vi "component orientation check.vi"(8 "error in":errorcluster, 10 "input cluster":T1, 11 "Gantry In":refnum<k24>) -> (0 "error out":errorcluster, 1 "Wrong Orientation?":bool, 2 "output cluster":T1, 3 "Gantry Out":refnum<k24>)   [LabVIEW 2021, in "Component Tray.lvclass"]
uses:
  Component Tray.lvclass
  Find Component.ctl
  Controller/Camera/Machine Vision.ctl
  C:/Program Files (x86)/Aerotech/A3200/LabVIEW/2010/Bin/Aerotech.A3200.dll
  Program Files (x86)/Aerotech/A3200/LabVIEW/2010/Bin/Aerotech.A3200.dll
  Controller/Motion/A3200/A3200.lvclass
  Controller/Camera/Camera.lvclass
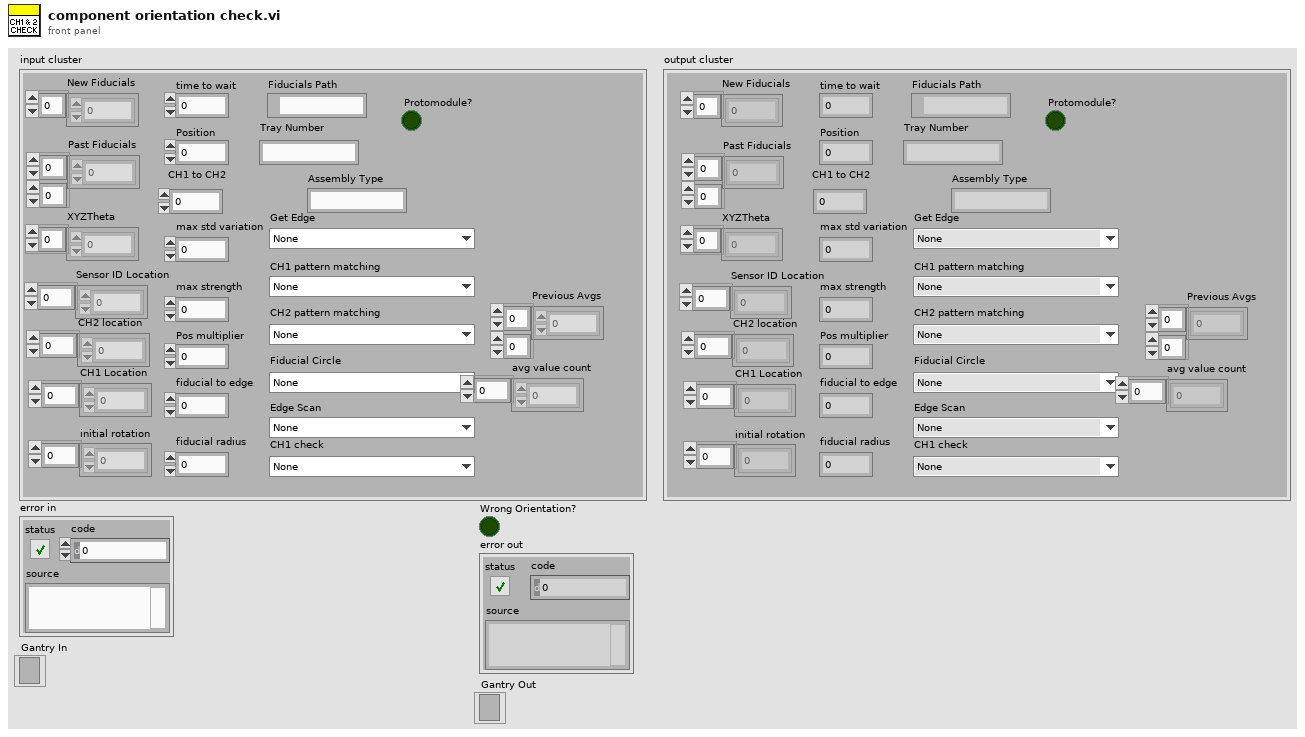
[diagram p1: front panel]
types:
  T1 = typedef "Component Tray.lvclass/Find Component.ctl" = cluster{"New Fiducials":dbl[], "Past Fiducials":dbl[][], "XYZTheta":dbl[], "Fiducials Path":path, "Position":i32, "CH1 Location":dbl[], "Sensor ID Location":dbl[], "initial rotation":dbl[], "CH2 location":dbl[], "max std variation":dbl, "max strength":dbl, "CH2 pattern matching":T2, "Fiducial Circle":T2, "Get Edge":T2, "Pos multiplier":dbl, "time to wait":u32, "fiducial to edge":dbl, "Protomodule?":bool, "Assembly Type":string, "CH1 to CH2":dbl, "Tray Number":string, "fiducial radius":dbl, "4 fiducials?":bool, "CH1 check":T2, "Edge Scan":T2, "CH1 pattern matching":T2, "Sensor Thickness":dbl, "Previous Avgs":dbl[][], "avg value count":dbl[]}
  T2 = typedef "Camera.lvclass/Machine Vision.ctl" = enum16{"None", "Assembly Tray Circle", "Assembly Tray Fiducial", "Partial Hexaboard", "sensor edge init", "HB edge init", "sensor edge pos1", "sensor edge pos2", "HB edge pos1", "HB edge pos2", "Sensor CH1-2", "HB CH1", "HB CH2", "V3 Sensor Circle", "Hexaboard Circle", "sensor CH1 check", "HB CH1 check ", "sensor ID"}
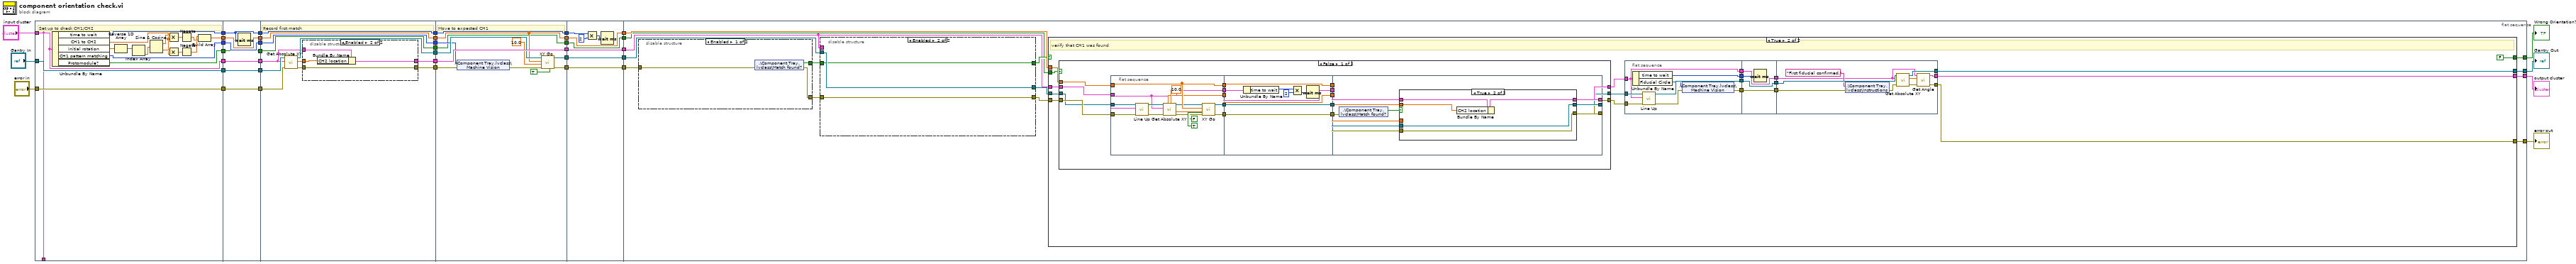
[diagram p0: block diagram]
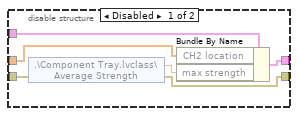
[diagram p2: hidden frame]
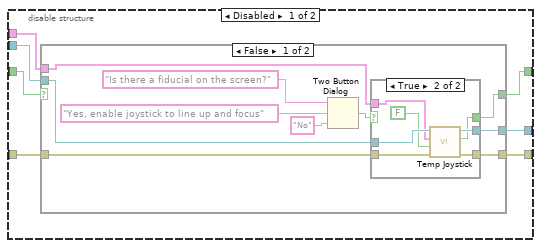
[diagram p3: hidden frame]
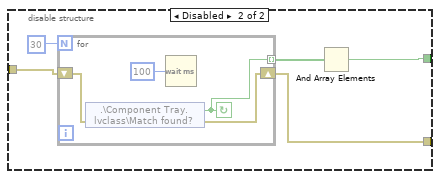
[diagram p6: hidden frame]
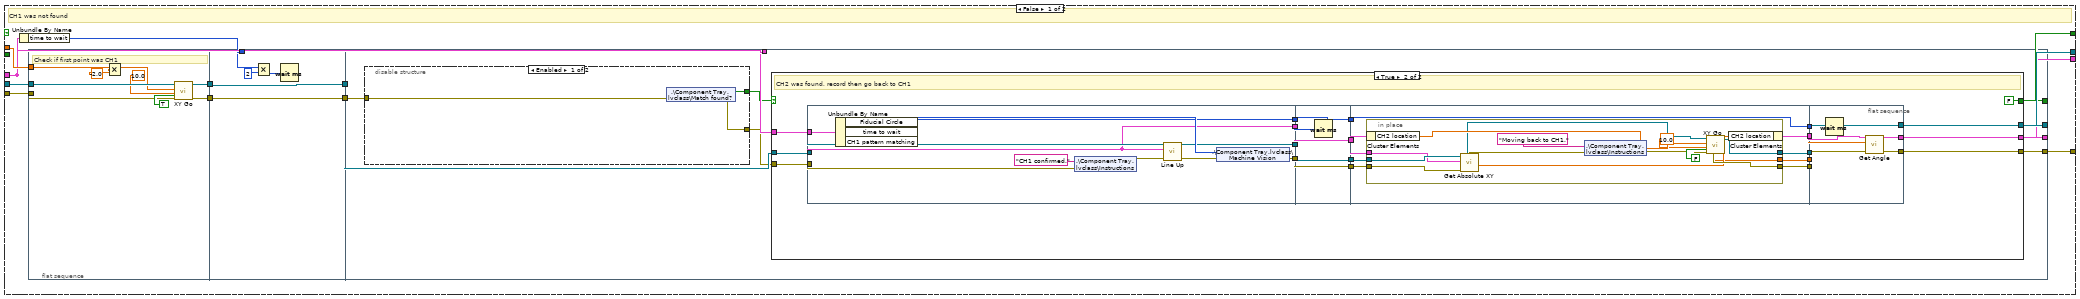
[diagram p7: hidden frame]
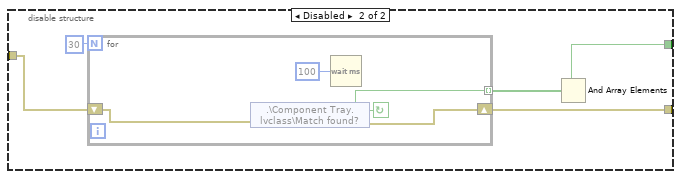
[diagram p8: hidden frame]
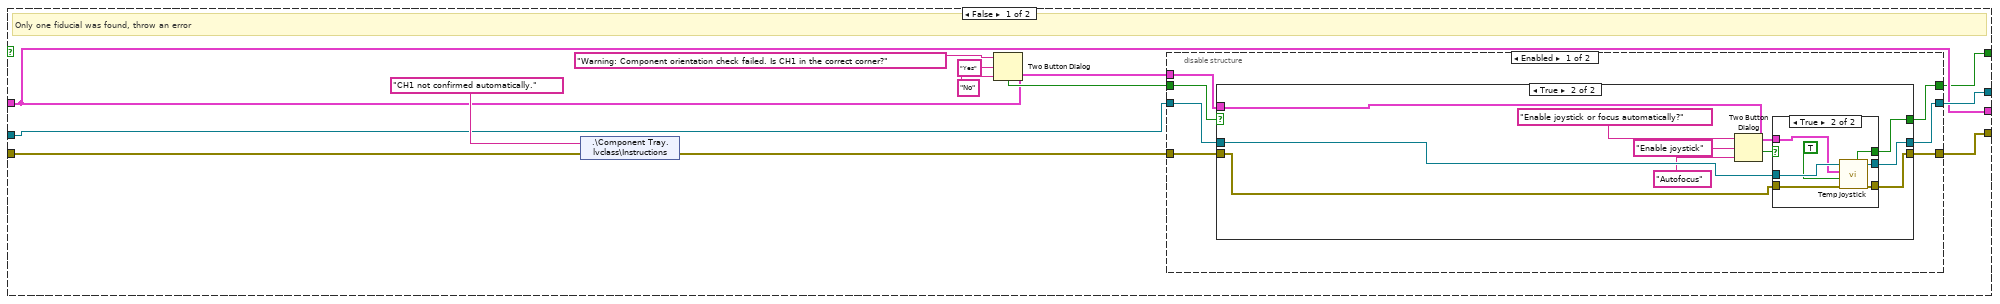
[diagram p9: hidden frame]
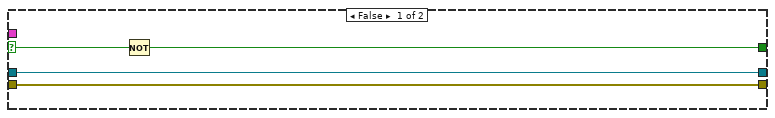
[diagram p10: hidden frame]
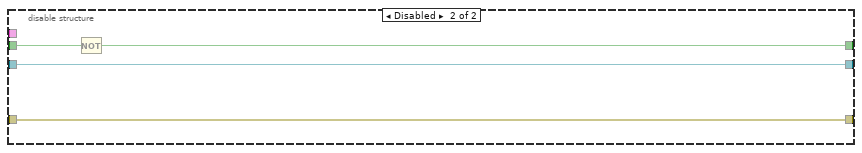
[diagram p12: hidden frame]
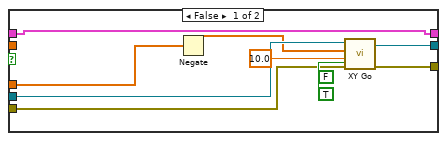
[diagram p13: hidden frame]
diagram:
  n1 = flat-sequence {
    tunnel: [w47] -> w32
    tunnel: [w46] -> w31
    tunnel: [w41] -> w30
    tunnel: [w56] -> w29
    tunnel: [w49] -> w28
    tunnel: [w48] -> w27
    tunnel: "input cluster" -> [w41]
    tunnel: "error in" -> [w46]
    tunnel: "Gantry In" -> [w47]
    tunnel: [w41] -> _
    tunnel: [w40] -> w1
    tunnel: w32 -> [w63]
    tunnel: [w63] -> w26
    tunnel: w31 -> [w62]
    tunnel: [w62] -> w25
    tunnel: w30 -> [w61]
    tunnel: [w61] -> w24
    tunnel: w29 -> [w60]
    tunnel: [w60] -> w23
    tunnel: w28 -> [w59]
    tunnel: [w59] -> w22
    tunnel: w27 -> [w58]
    tunnel: [w58] -> w21
    tunnel: [w57] -> w2
    tunnel: w1 -> [w57]
    tunnel: w26 -> [w74]
    tunnel: w25 -> [w73]
    tunnel: w24 -> [w65]
    tunnel: w23 -> [w68]
    tunnel: w22 -> [w71]
    tunnel: [w72] -> w20
    tunnel: [w66] -> w19
    tunnel: [w71] -> w18
    tunnel: [w70] -> w17
    tunnel: [w69] -> w16
    tunnel: w21 -> [w69]
    tunnel: [w68] -> w15
    tunnel: [w64] -> w3
    tunnel: w2 -> [w64]
    tunnel: w20 -> [w97]
    tunnel: w19 -> [w88]
    tunnel: w18 -> [w89]
    tunnel: w17 -> [w94]
    tunnel: w16 -> [w91]
    tunnel: [w92] -> w14
    tunnel: [w93] -> w13
    tunnel: [w97] -> w12
    tunnel: w15 -> [w90]
    tunnel: [w90] -> w11
    tunnel: [w89] -> w10
    tunnel: [w86] -> w4
    tunnel: w3 -> [w86]
    tunnel: w14 -> [w105]
    tunnel: [w105] -> w9
    tunnel: w13 -> [w104]
    tunnel: [w104] -> w8
    tunnel: w12 -> [w103]
    tunnel: [w103] -> w7
    tunnel: w11 -> [w101]
    tunnel: w10 -> [w102]
    tunnel: [w102] -> w6
    tunnel: [w98] -> w5
    tunnel: w4 -> [w98]
    tunnel: [w116] -> w33
    tunnel: [w118] -> w34
    tunnel: [w119] -> w39
    tunnel: w9 -> [w111]
    tunnel: w8 -> [w114]
    tunnel: w7 -> [w107]
    tunnel: w6 -> [w117]
    tunnel: [w115] -> w35
    tunnel: w5 -> [w106]
    frame #0 {
      # "Set up to check CH1/CH2"
      n2 = Unbundle By Name(w41) -> ("time to wait"=w56:u32, "CH1 to CH2"=w50:dbl, "initial rotation"=w51:dbl[], "CH1 pattern matching"=w48:T2, "Protomodule?"=w40:bool)
      n3 = Reverse 1D Array(array=w51) -> (reversed array=w52:dbl[])
      n4 = Index Array(array=w52) -> (element=w55:dbl)  [unwired: 1 in]
      n5 = Sine & Cosine(0:w55) -> (1:w54:dbl, 2:w53:dbl)
      n6 = Multiply(x=w54, y=w50) -> (x*y=w45:dbl)
      n7 = Multiply(x=w53, y=w50) -> (x*y=w43:dbl)
      n8 = Negate(x=w45) -> (-x=w44:dbl)
      n9 = Negate(x=w43) -> (-x=w42:dbl)
      n10 = Build Array(w42, w44) -> (w49:dbl[])
    }
    frame #1 {
      n11 = Wait (ms)(milliseconds to wait=w60) -> ()  [unwired: 1 out]
    }
    frame #2 {
      # "Record first match"
      n12 = call "Get Absolute XY.vi"("error in (no error)"=w73, "Component"=w65, "Gantry In"=w74) -> ("error out"=w67:errorcluster, "Abs XY"=w75:dbl[], "Gantry Out"=w70:refnum<k24>)  [unwired: 6 in]
      n13 = disable-structure shown="Enabled" {
        disable-tunnel: w65 -> [w81 w84]
        disable-tunnel: w75 -> [w80 w85]
        disable-tunnel: [w79 w83] -> w72
        disable-tunnel: w67 -> [w77 w82]
        disable-tunnel: [w76 w82] -> w66
        frame Disabled {
          n14 = shared-variable ".\\Component Tray.lvclass\\Average Strength"(error in=w77) -> (w78:dbl, error out=w76:errorcluster)
          n15 = Bundle By Name(cluster=w81, "CH2 location"=w80, "max strength"=w78) -> (w79:T1)
        }
        frame Enabled {
          n16 = Bundle By Name(cluster=w84, "CH2 location"=w85) -> (w83:T1)
        }
      }
    }
    frame #3 {
      # "Move to expected CH1"
      n17 = shared-variable ".\\Component Tray.lvclass\\Machine Vision"(w91, error in=w88) -> (error out=w87:errorcluster)
      n18 = call "XY Go.vi"("Increment?"=TRUE, "error in (no error)"=w87, "Speed"=10.0, "XY In"=w89, "Gantry In"=w94) -> ("error out"=w93:errorcluster, "Gantry Out"=w92:refnum<k24>)  [unwired: 4 in, 1 out]
    }
    frame #4 {
      n19 = Multiply(x=w101, y=u32 2) -> (x*y=w99:u32)
      n20 = Wait (ms)(milliseconds to wait=w99) -> ()  [unwired: 1 out]
    }
    frame #5 {
      n21 = disable-structure shown="Enabled" {
        disable-tunnel: [w155 w156] -> w113
        disable-tunnel: w114 -> [w154 w158]
        disable-tunnel: [w153 w157] -> w108
        frame Enabled {
          n22 = shared-variable ".\\Component Tray.lvclass\\Match found?"(error in=w154) -> (w155:bool, error out=w153:errorcluster)
        }
        frame Disabled {
          n23 = for {
            N: 30 -> [_]
            tunnel: [w161] -> w159 mode=indexing
            shift-right: [w162] -> w157
            shift-left: w158 -> [w163]
            stop <- w161 continue-if-true
            n24 = shared-variable ".\\Component Tray.lvclass\\Match found?"(error in=w163) -> (w161:bool, error out=w162:errorcluster)
            n25 = Wait (ms)(milliseconds to wait=u32 100) -> ()  [unwired: 1 out]
          }
          n26 = And Array Elements(Boolean array=w159) -> (logical AND=w156:bool)
        }
      }
      n27 = disable-structure shown="Enabled" {
        disable-tunnel: w113 -> [w126 w150]
        disable-tunnel: [w125 w150] -> w112
        disable-tunnel: w111 -> [w124 w151]
        disable-tunnel: [w123 w151] -> w110
        disable-tunnel: [w122 w152] -> w109
        disable-tunnel: w108 -> [w121 w152]
        disable-tunnel: w107 -> [w120 _]
        frame Disabled {
          n28 = case shown="False" w126 {
            selector: w126 -> [_ w149]
            tunnel: [w127 w149] -> w125
            tunnel: w124 -> [w132 w148]
            tunnel: [w131 w148] -> w123
            tunnel: [w130 w147] -> w122
            tunnel: w121 -> [w129 w147]
            tunnel: w120 -> [w128 _]
            frame False {
              n29 = Two Button Dialog(message="Is there a fiducial on the screen?", 1:"No" ("F button name (\"Cancel\")"), 2:"Yes, enable joystick to line up and focus" ("T button name (\"OK\")")) -> (T button?=w133:bool)
              n30 = case shown="True" w133 {
                selector: w133 -> [w137 _]
                tunnel: w132 -> [w139 w146]
                tunnel: [w139 w145] -> w131
                tunnel: [w138 w144] -> w130
                tunnel: w129 -> [w138 w143]
                tunnel: w128 -> [_ w141]
                tunnel: [w137 w140] -> w127
                frame False {
                }
                frame True {
                  n31 = call "Temp Joystick.vi"("error in (no error)"=w143, "Fiducial?"=FALSE ("Dialog?"), "Component"=w141, "Gantry In"=w146) -> ("error out"=w144:errorcluster, "Error?"=w140:bool, "Gantry Out"=w145:refnum<k24>)  [unwired: 5 in]
                }
              }
            }
            frame True {
            }
          }
        }
        frame Enabled {
        }
      }
      n32 = case shown="True" w112 {
        tunnel: w110 -> [w177 w326]
        tunnel: [w176 w340] -> w119
        tunnel: w109 -> [w175 w328]
        tunnel: [w174 w336] -> w118
        tunnel: w117 -> [w173 w330]
        tunnel: w107 -> [w172 w329]
        tunnel: [w170 w335] -> w116
        tunnel: [w171 FALSE] -> w115
        tunnel: w106 -> [_ w327]
        frame False {
          # "CH1 was not found"
          n33 = Unbundle By Name(w172) -> ("time to wait"=w165:u32)
          n34 = flat-sequence {
            tunnel: w177 -> [w186]
            tunnel: w175 -> [w183]
            tunnel: w173 -> [w180]
            tunnel: [w185] -> w169
            tunnel: [w182] -> w167
            tunnel: w169 -> [w191]
            tunnel: [w191] -> w168
            tunnel: w167 -> [w190]
            tunnel: [w190] -> w166
            tunnel: w165 -> [w189]
            tunnel: [w198] -> w174
            tunnel: [w199] -> w176
            tunnel: w168 -> [w200]
            tunnel: w166 -> [w195]
            tunnel: [w192] -> w171
            tunnel: w172 -> [w197]
            tunnel: [w196] -> w170
            frame #0 {
              # "Check if first point was CH1"
              n35 = Multiply(x=w180, y=-2.0) -> (x*y=w179:dbl[])
              n36 = call "XY Go.vi"("Increment?"=TRUE, "error in (no error)"=w183, "Speed"=10.0, "XY In"=w179, "Gantry In"=w186) -> ("error out"=w182:errorcluster, "Gantry Out"=w185:refnum<k24>)  [unwired: 4 in, 1 out]
            }
            frame #1 {
              n37 = Multiply(x=w189, y=u32 2) -> (x*y=w187:u32)
              n38 = Wait (ms)(milliseconds to wait=w187) -> ()  [unwired: 1 out]
            }
            frame #2 {
              n39 = disable-structure shown="Enabled" {
                disable-tunnel: w195 -> [w203 w206]
                disable-tunnel: [w202 w205] -> w194
                disable-tunnel: [w201 w204] -> w193
                frame Enabled {
                  n40 = shared-variable ".\\Component Tray.lvclass\\Match found?"(error in=w203) -> (w201:bool, error out=w202:errorcluster)
                }
                frame Disabled {
                  n41 = for {
                    N: 30 -> [_]
                    tunnel: [w209] -> w207 mode=indexing
                    shift-right: [w210] -> w205
                    shift-left: w206 -> [w211]
                    stop <- w209 continue-if-true
                    n42 = shared-variable ".\\Component Tray.lvclass\\Match found?"(error in=w211) -> (w209:bool, error out=w210:errorcluster)
                    n43 = Wait (ms)(milliseconds to wait=u32 100) -> ()  [unwired: 1 out]
                  }
                  n44 = And Array Elements(Boolean array=w207) -> (logical AND=w204:bool)
                }
              }
              n45 = case shown="True" w193 {
                tunnel: w200 -> [w215 w279]
                tunnel: [w216 w278] -> w199
                tunnel: w194 -> [w223 w277]
                tunnel: [w222 w262] -> w198
                tunnel: w197 -> [w214 w276]
                tunnel: [w214 w261] -> w196
                tunnel: [w213 FALSE ("Error?")] -> w192
                frame False {
                  # "Only one fiducial was found, throw an error"
                  n46 = shared-variable ".\\Component Tray.lvclass\\Instructions"("CH1 not confirmed automatically." ("Instructions"), error in=w223) -> (error out=w221:errorcluster)
                  n47 = Two Button Dialog(message="Warning: Component orientation check failed. Is CH1 in the correct corner?", 1:"No" ("F button name (\"Cancel\")"), 2:"Yes" ("T button name (\"OK\")")) -> (T button?=w217:bool)
                  n48 = disable-structure shown="Enabled" {
                    disable-tunnel: [w231 w259] -> w222
                    disable-tunnel: w221 -> [w230 w259]
                    disable-tunnel: w217 -> [w229 w257]
                    disable-tunnel: [w228 w258] -> w216
                    disable-tunnel: w215 -> [w227 w258]
                    disable-tunnel: w214 -> [w226 _]
                    disable-tunnel: [w225 w256] -> w213
                    frame Enabled {
                      n49 = case shown="True" w229 {
                        selector: w229 -> [w233 _]
                        tunnel: w227 -> [w235 w245]
                        tunnel: [w235 w244] -> w228
                        tunnel: [w234 w243] -> w231
                        tunnel: w230 -> [w234 w242]
                        tunnel: w226 -> [_ w241]
                        tunnel: [w232 w240] -> w225
                        frame False {
                          n50 = Not(x=w233) -> (.not. x?=w232:bool)
                        }
                        frame True {
                          n51 = Two Button Dialog(message="Enable joystick or focus automatically?", 1:"Autofocus" ("F button name (\"Cancel\")"), 2:"Enable joystick" ("T button name (\"OK\")")) -> (T button?=w236:bool)
                          n52 = case shown="True" w236 {
                            selector: w236 -> [w246 _]
                            tunnel: w245 -> [w248 w255]
                            tunnel: [w248 w254] -> w244
                            tunnel: [w247 w253] -> w243
                            tunnel: w242 -> [w247 w252]
                            tunnel: w241 -> [_ w250]
                            tunnel: [w246 w249] -> w240
                            frame False {
                            }
                            frame True {
                              n53 = call "Temp Joystick.vi"("error in (no error)"=w252, "Fiducial?"=TRUE ("Dialog?"), "Component"=w250, "Gantry In"=w255) -> ("error out"=w253:errorcluster, "Error?"=w249:bool, "Gantry Out"=w254:refnum<k24>)  [unwired: 5 in]
                            }
                          }
                        }
                      }
                    }
                    frame Disabled {
                      n54 = Not(x=w257) -> (.not. x?=w256:bool)
                    }
                  }
                }
                frame True {
                  # "CH2 was found, record then go back to CH1"
                  n55 = flat-sequence {
                    tunnel: w276 -> [w280]
                    tunnel: [w283] -> w271
                    tunnel: [w288] -> w269
                    tunnel: [w287] -> w267
                    tunnel: [w280] -> w265
                    tunnel: w277 -> [w285]
                    tunnel: w279 -> [w284]
                    tunnel: w271 -> [w293]
                    tunnel: [w293] -> w270
                    tunnel: w269 -> [w292]
                    tunnel: [w292] -> w268
                    tunnel: w267 -> [w291]
                    tunnel: [w291] -> w266
                    tunnel: w265 -> [w290]
                    tunnel: [w290] -> w264
                    tunnel: [w298] -> w275
                    tunnel: [w299] -> w274
                    tunnel: [w300] -> w273
                    tunnel: [w301] -> w272
                    tunnel: w264 -> [w295]
                    tunnel: w266 -> [w296]
                    tunnel: w268 -> [w301]
                    tunnel: w270 -> [w297]
                    tunnel: [w294] -> w260
                    tunnel: [w322] -> w278
                    tunnel: w275 -> [w322]
                    tunnel: w274 -> [w320]
                    tunnel: w273 -> [w319]
                    tunnel: w272 -> [w321]
                    tunnel: [w318] -> w262
                    tunnel: [w317] -> w261
                    tunnel: w260 -> [w316]
                    frame #0 {
                      n56 = Unbundle By Name(w280) -> ("Fiducial Circle"=w289:T2, "time to wait"=w288:u32)  [unwired: 1 out]
                      n57 = shared-variable ".\\Component Tray.lvclass\\Instructions"("CH1 confirmed." ("Instructions"), error in=w285) -> (error out=w281:errorcluster)
                      n58 = call "Line Up.vi"("error IO"=w281, "Component"=w280, "Gantry In"=w284) -> ("error out"=w282:errorcluster, "Gantry Out"=w283:refnum<k24>)  [unwired: 6 in, 1 out]
                      n59 = shared-variable ".\\Component Tray.lvclass\\Machine Vision"(w289, error in=w282) -> (error out=w287:errorcluster)
                    }
                    frame #1 {
                      n60 = Wait (ms)(milliseconds to wait=w292) -> ()  [unwired: 1 out]
                    }
                    frame #2 {
                      n61 = in-place {
                        in-place-border: [w302] -> w294
                        in-place-border: [w314] -> w299
                        in-place-border: [w313] -> w298
                        in-place-border: w297 -> [w306]
                        in-place-border: w296 -> [w305]
                        in-place-border: w295 -> [w304]
                        n62 = in-place-cluster #1(w295) -> ("CH2 location"=w315:dbl[])
                        n63 = call "Get Absolute XY.vi"("error in (no error)"=w305, "Component"=w304, "Gantry In"=w306) -> ("error out"=w308:errorcluster, "Abs XY"=w311:dbl[], "Gantry Out"=w310:refnum<k24>)  [unwired: 6 in]
                        n64 = shared-variable ".\\Component Tray.lvclass\\Instructions"("Moving back to CH1." ("Instructions"), error in=w308) -> (error out=w307:errorcluster)
                        n65 = call "XY Go.vi"("Increment?"=FALSE, "error in (no error)"=w307, "Speed"=10.0, "XY In"=w315, "Gantry In"=w310) -> ("error out"=w314:errorcluster, "XY Out"=w302:dbl[], "Gantry Out"=w313:refnum<k24>)  [unwired: 4 in]
                        n66 = in-place-cluster #1("CH2 location"=w311) -> (w300:T1)
                      }
                    }
                    frame #3 {
                      n67 = Wait (ms)(milliseconds to wait=w321) -> ()  [unwired: 1 out]
                      n68 = call "Get Angle.vi"("error in"=w320, "array"=w316, "input cluster"=w319) -> ("error out"=w318:errorcluster, "output cluster"=w317:T1)  [unwired: 7 in]
                    }
                  }
                }
              }
            }
          }
        }
        frame True {
          # "verify that CH1 was found"
          n69 = case shown="False" w327 {
            tunnel: w330 -> [w348 _]
            tunnel: w329 -> [w347 w407]
            tunnel: w328 -> [w346 w405]
            tunnel: w326 -> [w345 w406]
            tunnel: [w344 w407] -> w325
            tunnel: [w343 w406] -> w324
            tunnel: [w342 w405] -> w323
            frame False {
              n70 = flat-sequence {
                tunnel: w345 -> [w368]
                tunnel: w348 -> [w365]
                tunnel: w346 -> [w367]
                tunnel: [w369] -> w358
                tunnel: w347 -> [w359]
                tunnel: [w366] -> w357
                tunnel: [w365] -> w356
                tunnel: [w359] -> w355
                tunnel: [w360] -> w354
                tunnel: w358 -> [w378]
                tunnel: [w378] -> w353
                tunnel: w357 -> [w377]
                tunnel: [w377] -> w352
                tunnel: w356 -> [w376]
                tunnel: [w376] -> w351
                tunnel: w355 -> [w374]
                tunnel: [w374] -> w350
                tunnel: [w375] -> w349
                tunnel: w354 -> [w375]
                tunnel: w353 -> [w387]
                tunnel: w352 -> [w388]
                tunnel: w351 -> [w386]
                tunnel: w350 -> [w385]
                tunnel: w349 -> [w384]
                tunnel: [w383] -> w344
                tunnel: [w382] -> w343
                tunnel: [w381] -> w342
                frame #0 {
                  n71 = call "Line Up.vi"("error IO"=w367, "Component"=w359, "Gantry In"=w368) -> ("error out"=w362:errorcluster, "Gantry Out"=w364:refnum<k24>)  [unwired: 6 in, 1 out]
                  n72 = call "Get Absolute XY.vi"("error in (no error)"=w362, "Component"=w359, "Gantry In"=w364) -> ("error out"=w361:errorcluster, "Abs XY"=w360:dbl[], "Gantry Out"=w363:refnum<k24>)  [unwired: 6 in]
                  n73 = call "XY Go.vi"("Increment?"=TRUE, "return immediately"=FALSE, "error in (no error)"=w361, "Speed"=10.0, "XY In"=w365, "Gantry In"=w363) -> ("error out"=w369:errorcluster, "Gantry Out"=w366:refnum<k24>)  [unwired: 3 in, 1 out]
                }
                frame #1 {
                  n74 = Unbundle By Name(w374) -> ("time to wait"=w373:u32)
                  n75 = Multiply(x=w373, y=u32 2) -> (x*y=w379:u32)
                  n76 = Wait (ms)(milliseconds to wait=w379) -> ()  [unwired: 1 out]
                }
                frame #2 {
                  n77 = shared-variable ".\\Component Tray.lvclass\\Match found?"(error in=w387) -> (w389:bool)  [unwired: 1 out]
                  n78 = case shown="True" w389 {
                    tunnel: w388 -> [w396 w401]
                    tunnel: w387 -> [w395 w400]
                    tunnel: w386 -> [w394 _]
                    tunnel: w385 -> [w390 w404]
                    tunnel: w384 -> [_ w403]
                    tunnel: [w392 w401] -> w382
                    tunnel: [w391 w400] -> w381
                    tunnel: [w390 w402] -> w383
                    frame False {
                      n79 = Negate(x=w394) -> (-x=w393:dbl[])
                      n80 = call "XY Go.vi"("Increment?"=TRUE, "return immediately"=FALSE, "error in (no error)"=w395, "Speed"=10.0, "XY In"=w393, "Gantry In"=w396) -> ("error out"=w391:errorcluster, "Gantry Out"=w392:refnum<k24>)  [unwired: 3 in, 1 out]
                    }
                    frame True {
                      n81 = Bundle By Name(cluster=w404, "CH2 location"=w403) -> (w402:T1)
                    }
                  }
                }
              }
            }
            frame True {
            }
          }
          n82 = flat-sequence {
            tunnel: [w413] -> w334
            tunnel: [w414] -> w333
            tunnel: [w409] -> w332
            tunnel: [w410] -> w331
            tunnel: w325 -> [w410]
            tunnel: w324 -> [w412]
            tunnel: w323 -> [w411]
            tunnel: w334 -> [w419]
            tunnel: [w419] -> w339
            tunnel: w333 -> [w418]
            tunnel: [w418] -> w338
            tunnel: w332 -> [w417]
            tunnel: w331 -> [w416]
            tunnel: [w416] -> w337
            tunnel: [w428] -> w340
            tunnel: w339 -> [w429]
            tunnel: w338 -> [w427]
            tunnel: w337 -> [w420]
            tunnel: [w422] -> w336
            tunnel: [w421] -> w335
            frame #0 {
              n83 = Unbundle By Name(w410) -> ("time to wait"=w409:u32, "Fiducial Circle"=w408:T2)
              n84 = call "Line Up.vi"("error IO"=w411, "Component"=w410, "Gantry In"=w412) -> ("error out"=w415:errorcluster, "Gantry Out"=w413:refnum<k24>)  [unwired: 6 in, 1 out]
              n85 = shared-variable ".\\Component Tray.lvclass\\Machine Vision"(w408, error in=w415) -> (error out=w414:errorcluster)
            }
            frame #1 {
              n86 = Wait (ms)(milliseconds to wait=w417) -> ()  [unwired: 1 out]
            }
            frame #2 {
              n87 = shared-variable ".\\Component Tray.lvclass\\Instructions"("First fiducial confirmed." ("Instructions"), error in=w427) -> (error out=w425:errorcluster)
              n88 = call "Get Absolute XY.vi"("error in (no error)"=w425, "Component"=w420, "Gantry In"=w429) -> ("error out"=w424:errorcluster, "Abs XY"=w423:dbl[], "Gantry Out"=w428:refnum<k24>)  [unwired: 6 in]
              n89 = call "Get Angle.vi"("error in"=w424, "array"=w423, "input cluster"=w420) -> ("error out"=w422:errorcluster, "output cluster"=w421:T1)  [unwired: 7 in]
            }
          }
        }
      }
    }
  }
  "Wrong Orientation?" <- w35
  "output cluster" <- w33
  "error out" <- w34
  "Gantry Out" <- w39
